vi "2ndhitter.vi"(2 "Marble Req":dbl, 3 "NXT/EV3":T1) -> (0 "NXT/EV3 2":T1)   [LabVIEW 2016]
uses:
  <vilib>/NXT/Subs/LVHSConnector.ctl
  <vilib>/NXT/LegoClasses/BrickReference/BrickReference.lvclass
  <vilib>/NXT/Block Support/NXT_OutputPort.ctl
  <vilib>/NXT/NXTIO Xnodes/NXTIONodeSubVIs/NXTMotorRunDistance.vi
  <vilib>/NXT/Dual Mode Library/Waits/Wait_Num.vi
  <vilib>/NXT/NXTIO Xnodes/AddressXNode/NXTIOAddress.xnode
  <vilib>/NXT/NXTIO Xnodes/NXTIOXNode/NXTIO.xnode
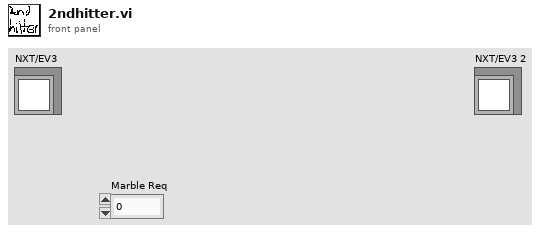
[diagram p1: front panel]
types:
  T1 = typedef "LVHSConnector.ctl" = refnum<class "BrickReference.lvclass">
  T2 = typedef "NXT_OutputPort.ctl" = u8
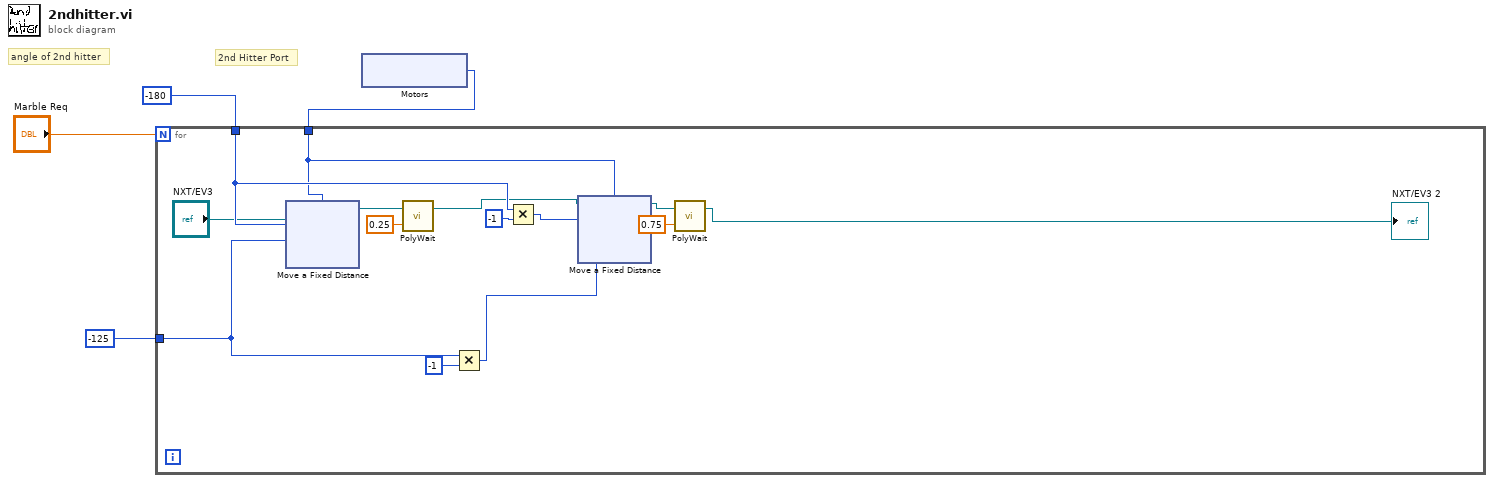
[diagram p0: block diagram]
diagram:
  # "angle of 2nd hitter"
  # "2nd Hitter Port"
  n1 = xnode "Motors"() -> ("Motor"=w4:T2)
  n2 = for {
    N: "Marble Req" -> [_]
    tunnel: w4 -> [w12]
    tunnel: -180 -> [w16]
    tunnel: -125 -> [w10]
    n3 = xnode "Move a Fixed Distance"("Speed 1"=w10, "Distance 1"=w16, "Motors"=w12, "NXT/EV3"="NXT/EV3") -> ("NXT/EV3"=w17:T1)
    n4 = call-poly <vilib>:"PolyWait.vi"("Time (1 sec)"=sgl 0.25, "NXT/EV3"=w17) -> ("NXT/EV3"=w13:T1)  [unwired: 2 in]
    n5 = Multiply(x=w10, y=-1) -> (x*y=w9:i32)
    n6 = Multiply(x=w16, y=-1) -> (x*y=w14:i32)
    n7 = xnode "Move a Fixed Distance"("Speed 1"=w9, "Distance 1"=w14, "Motors"=w12, "NXT/EV3"=w13) -> ("NXT/EV3"=w7:T1)
    n8 = call-poly <vilib>:"PolyWait.vi"("Time (1 sec)"=sgl 0.75, "NXT/EV3"=w7) -> ("NXT/EV3"=→"NXT/EV3 2":T1)  [unwired: 2 in]
  }
